vi "Simulate GPS Logfile (Keith Koch's conflicted copy 2013-05-10).vi"(1 "file path (dialog if empty)":path=path "C:/Users/ATV Project/Dropbox/Auto-Steering and Obstacle Avoidance System Project/Software/VI's/_Data/Log_Files(GPS)/GPS_LOG_5-6-2013_6-12 PM") -> (0 "Time(s)":i32)   [LabVIEW 2011]
uses:
  _GlobalVariables&Libraries/ATV Program Global Variables.vi
  <vilib>/Utility/file.llb/Read From Spreadsheet File (DBL).vi
panel:
  in  "Plot Delay":u32=500
  out "Duration(s)":i32
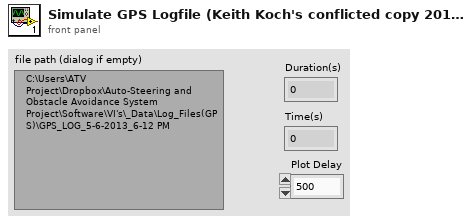
[diagram p1: front panel]
types:
  T1 = cluster{"Navigation Coordinates":cluster{"Latitude":dbl, "Longitude":dbl}[], "Coordinate Count":u32, "Drive Speed":string, "Steer Angle":dbl, "Steering":dbl, "Direction to next Coordinate":dbl, "Drive":dbl, "Navigation Path":string}
  T2 = cluster{"End ATV Program":bool, "E-Stop":bool, "Save Logfile":bool, "Logfile Iteration Delay (ms)":u32, "Loop iteration time (ms)":u32, "Logfile Location":path, "Default GPS Navigation Path":path, "Computer":string, "Default GPS Boundary Path":path}
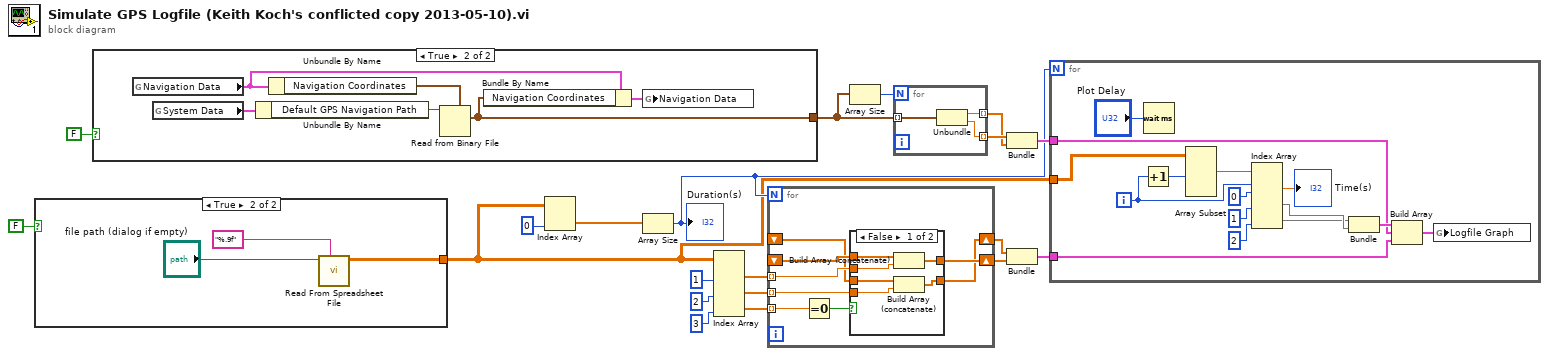
[diagram p0: block diagram]
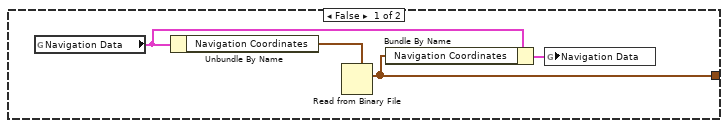
[diagram p2: hidden frame]
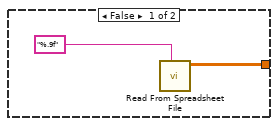
[diagram p3: hidden frame]
diagram:
  n1 = case shown="True" FALSE {
    tunnel: [w21 w23] -> w6
    frame False {
      n2 = call-poly <vilib>:"Read From Spreadsheet File.vi"("format (%.3f)"="%.9f") -> ("all rows"=w21:dbl[][])  [unwired: 6 in, 4 out]
    }
    frame True {
      n3 = call-poly <vilib>:"Read From Spreadsheet File.vi"("format (%.3f)"="%.9f", "file path (dialog if empty)"="file path (dialog if empty)") -> ("all rows"=w23:dbl[][])  [unwired: 5 in, 4 out]
    }
  }
  n4 = case shown="True" FALSE {
    tunnel: [w26 w32] -> w4
    frame False {
      n5 = global read "ATV Program Global Variables.vi" "Navigation Data"() -> (w27:T1)
      n6 = Unbundle By Name(w27) -> ("Navigation Coordinates"=w29:cluster{"Latitude":dbl, "Longitude":dbl}[])
      n7 = Read from Binary File(5:w29) -> (2:w26:cluster{"Latitude":dbl, "Longitude":dbl}[])  [unwired: 5 in, 3 out]
      n8 = Bundle By Name(cluster=w27, "Navigation Coordinates"=w26) -> (w28:T1)
      n9 = global write "ATV Program Global Variables.vi" "Navigation Data"(w28) -> ()
    }
    frame True {
      n10 = global read "ATV Program Global Variables.vi" "Navigation Data"() -> (w33:T1)
      n11 = global read "ATV Program Global Variables.vi" "System Data"() -> (w31:T2)
      n12 = Unbundle By Name(w31) -> ("Default GPS Navigation Path"=w30:path)
      n13 = Unbundle By Name(w33) -> ("Navigation Coordinates"=w35:cluster{"Latitude":dbl, "Longitude":dbl}[])
      n14 = Read from Binary File(5:w35, 11:w30) -> (2:w32:cluster{"Latitude":dbl, "Longitude":dbl}[])  [unwired: 4 in, 3 out]
      n15 = Bundle By Name(cluster=w33, "Navigation Coordinates"=w32) -> (w34:T1)
      n16 = global write "ATV Program Global Variables.vi" "Navigation Data"(w34) -> ()
    }
  }
  n17 = Index Array(array=w6, index (col)=0) -> (element=w15:dbl[])  [unwired: 1 in]
  n18 = Array Size(array=w15) -> (size(s)=w7:i32)
  "Duration(s)" <- w7
  n19 = Index Array(array=w6, index (col) #1=1 ("index (col)"), index (col) #2=2 ("index (col)"), index (col) #3=3 ("index (col)")) -> (element #1=w10:dbl[], element #2=w9:dbl[], element #3=w11:dbl[])  [unwired: 3 in]
  n20 = for {
    N: w7 -> [_]
    tunnel: w11 -> [w43] mode=indexing
    tunnel: w10 -> [w38] mode=indexing
    tunnel: w9 -> [w39] mode=indexing
    shift-right: [w41] -> w2
    shift-left: _ -> [w40]
    shift-right: [w37] -> w1
    shift-left: _ -> [w36]
    n21 = Equal To 0?(x=w43) -> (x = 0?=w42:bool)
    n22 = case shown="False" w42 {
      tunnel: [w47 w51] -> w41
      tunnel: w40 -> [w44 w51]
      tunnel: w39 -> [w48 _]
      tunnel: w38 -> [w49 _]
      tunnel: [w46 w50] -> w37
      tunnel: w36 -> [w45 w50]
      frame False {
        n23 = Build Array (concatenate)(w44, w49) -> (w47:dbl[])
        n24 = Build Array (concatenate)(w45, w48) -> (w46:dbl[])
      }
      frame True {
      }
    }
  }
  n25 = Array Size(array=w4) -> (size(s)=w20:i32)
  n26 = for {
    N: w20 -> [_]
    tunnel: w4 -> [w54] mode=indexing
    tunnel: [w53] -> w18 mode=indexing
    tunnel: [w52] -> w19 mode=indexing
    n27 = Unbundle(w54) -> ("Latitude"=w53:dbl, "Longitude"=w52:dbl)
  }
  n28 = Bundle(w19, w18) -> (w17:cluster{dbl[], dbl[]})  [unwired: 1 in]
  n29 = Bundle(w1, w2) -> (w8:cluster{dbl[], dbl[]})  [unwired: 1 in]
  n30 = for {
    N: w7 -> [_]
    tunnel: w17 -> [w63]
    tunnel: w6 -> [w60]
    tunnel: w8 -> [w55]
    i -> [w56]
    n31 = Increment(x=w56) -> (x+1=w57:i32)
    n32 = Wait (ms)(milliseconds to wait="Plot Delay") -> ()  [unwired: 1 out]
    n33 = Array Subset(array=w60, length (row)=w57) -> (w61:dbl[][])  [unwired: 3 in]
    n34 = Index Array(array=w61, index (row) #1=w56, index (col) #1=0 ("disabled index (col)"), index (col) #2=1 ("index (col)"), index (col) #3=2 ("index (col)")) -> (element #1=→"Time(s)":dbl, element #2=w66:dbl[], element #3=w65:dbl[])  [unwired: 2 in]
    n35 = Bundle(w65, w66) -> (w64:cluster{dbl[], dbl[]})  [unwired: 1 in]
    n36 = Build Array(w64, w63, w55) -> (w62:cluster{dbl[], dbl[]}[])
    n37 = global write "ATV Program Global Variables.vi" "Logfile Graph"(w62) -> ()
  }
